vi "iRobot Deinitialize.vi"(8 "error in":errorcluster, 11 "UART port in":T1) -> (0 "error out":errorcluster)   [LabVIEW 2010]
doc: "Stops wheels, clears UART, sets to safe mode, resets to standard baud rate, and terminates UART connection.\n\nThis VI both writes to AND reads from the serial port."
uses:
  UART/UART Port Type.ctl
  Actuator/Actuator Controls/iRobot LED.ctl
  Command/Command Controls/iRobot Baud.ctl
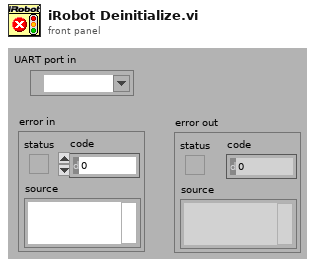
[diagram p1: front panel]
types:
  T1 = typedef "UART Port Type.ctl" = refnum<visa-resource-name>
  T2 = typedef "iRobot Baud.ctl" = enum8{"300", "600", "1200", "2400", "4800", "9600", "14400", "19200", "28800", "38400", "57600", "115200"}
  T3 = typedef "iRobot LED.ctl" = u8
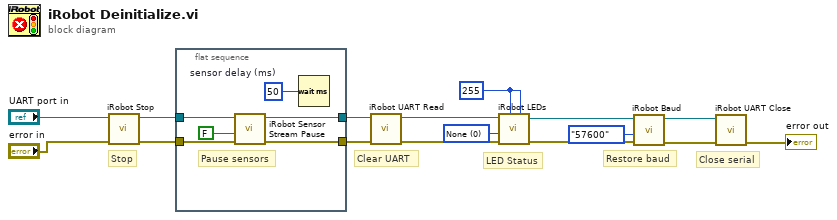
[diagram p0: block diagram]
diagram:
  w13 = T3 0 items=["None"=0, "Advance"=8, "Play"=2, "Advance + Play"=10] ("LEDs on")
  w1 = u8 255 ("Power LED Color (R-G)")
  # "Close serial"
  # "Restore baud"
  # "Clear UART"
  # "Stop"
  # "LED Status"
  n1 = call "iRobot Stop.vi"("error in"="error in", "UART port in"="UART port in") -> ("error out"=w7:errorcluster, "UART port out"=w15:T1)  [unwired: 8 out]
  n2 = flat-sequence {
    tunnel: w15 -> [w21]
    tunnel: [w19] -> w14
    tunnel: w7 -> [w18]
    tunnel: [w17] -> w6
    frame #0 {
      w20 = u32 50  # sensor delay (ms)
      # "Pause sensors"
      n3 = call "iRobot Sensor Stream Pause.vi"("error in"=w18, "Resume?"=FALSE, "UART port in"=w21) -> ("error out"=w17:errorcluster, "UART port out"=w19:T1)  [unwired: 1 in, 6 out]
      n4 = Wait (ms)(milliseconds to wait=w20) -> ()  [unwired: 1 out]
    }
  }
  n5 = call "iRobot UART Read.vi"("error in"=w6, "UART port in"=w14) -> ("error out"=w5:errorcluster, "UART port out"=w10:T1)  [unwired: 8 out]
  n6 = call "iRobot LEDs.vi"("Power LED Intensity (0-255)"=w1, "Power LED Color (G[0]-R[255])"=w1, "error in"=w5, "LEDs on"=w13, "UART port in"=w10) -> ("error out"=w4:errorcluster, "UART port out"=w12:T1)  [unwired: 2 in, 3 out]
  n7 = call "iRobot Baud.vi"("error in"=w4, "Baud Rate (BPS)"=iRobot_Baud."57600", "UART port in"=w12) -> ("error out"=w3:errorcluster, "UART port out"=w9:T1)  [unwired: 7 out]
  n8 = call "iRobot UART Close.vi"("error in"=w3, "UART port in"=w9) -> ("error out"=→"error out":errorcluster)  [unwired: 9 out]
